vi "SetTitle.vi"(0 "reference in":refnum<class "GUI.lvclass">, 11 "error in (no error)":errorcluster) -> (4 "reference out":refnum<class "GUI.lvclass">, 15 "error out":errorcluster)   [LabVIEW 2019, in "GUI.lvclass"]
uses:
  GUI.lvclass
  GUI.lvclass/GUI.ctl
panel:
  in  "Front Panel Window:Title":string
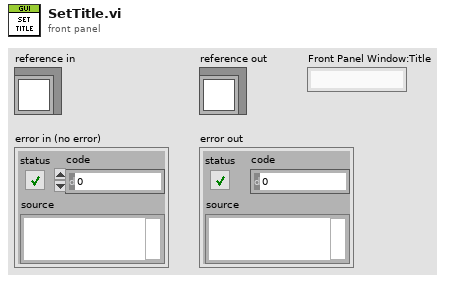
[diagram p1: front panel]
types:
  T1 = typedef "GUI.lvclass/Shered Data.ctl" = cluster{"WindowsState":T2, "UI VI":refnum<vi>, "SubPnl":refnum<vi>}
  T2 = typedef "GUI.lvclass/WindowsState.ctl" = enum16{"NotReady", "Ready", "Inserted", "Opened"}
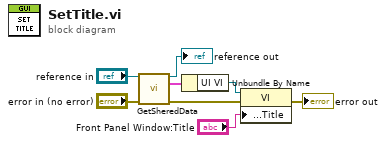
[diagram p0: block diagram]
diagram:
  n1 = call "GetSheredData.vi"("reference in"="reference in", "error in (no error)"="error in (no error)") -> ("reference out"=→"reference out":refnum<class "GUI.lvclass">, "data"=w7:T1, "error out"=w4:errorcluster)  [unwired: 11 in]
  n2 = Unbundle By Name(w7) -> ("UI VI"=w6:refnum<vi>)
  n3 = property class="VI"(reference=w6, error in=w4, "Front Panel.Title"="Front Panel Window:Title") -> (error out=→"error out":errorcluster)  [unwired: 1 out]
